vi "Get Log File Archive Location.vi"(8 "error in (no error)":errorcluster, 11 "log file in":T1 format="%.0x") -> (0 "error out":errorcluster, 1 "archive directory parts":string[](array[string]), 2 "archive closed log files":bool, 3 "log file out":T1 format="%.0x")   [LabVIEW 2027, in "Embedded Data Logger Scripting.lvlib"]
uses:
  Embedded Data Logger Scripting.lvlib
  <vilib>/NI VeriStand/Custom Device API/Custom Device Item Ref.ctl
  Shared/Constants.vi
  <vilib>/NI VeriStand/Custom Device API/Get Item Property (Boolean).vi
  <vilib>/NI VeriStand/Custom Device API/Get Item Property (String Array).vi
  <vilib>/NI VeriStand/Custom Device API/Custom Device API.lvlib
  Shared/Embedded Data Logger Shared.lvlib
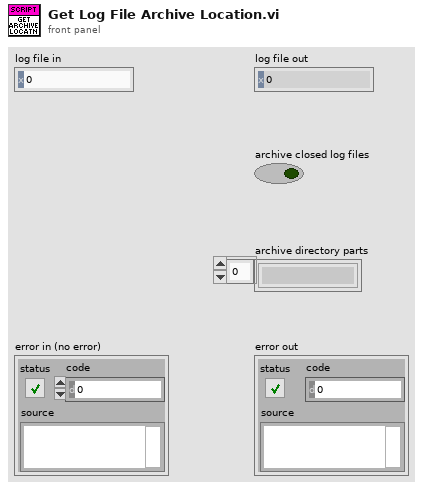
[diagram p1: front panel]
types:
  T1 = typedef "Custom Device API.lvlib/Custom Device Item Ref.ctl" = u64
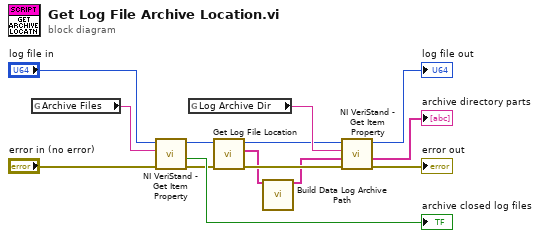
[diagram p0: block diagram]
diagram:
  n1 = global read "Constants.vi" "Archive Files"() -> (w7:string)
  n2 = call-poly <vilib>:"NI VeriStand - Get Item Property.vi"("error in (no error)"="error in (no error)", "Property Name"=w7, "Item Ref in"="log file in") -> ("error out"=w6:errorcluster, "Value"=→"archive closed log files":bool, "Item Ref out"=w5:T1)  [unwired: 1 in, 5 out]
  n3 = global read "Constants.vi" "Log Archive Dir"() -> (w14:string)
  n4 = call "Get Log File Location.vi"("error in (no error)"=w6, "log file in"=w5) -> ("error out"=w3:errorcluster, "directory parts"=w2:string[], "log file out"=w4:T1)  [unwired: 4 in, 3 out]
  n5 = call "Build Data Log Archive Path.vi"("Log Directory String Array"=w2) -> ("Log Archive Directory String Array"=w1:string[])  [unwired: 14 in]
  n6 = call-poly <vilib>:"NI VeriStand - Get Item Property.vi"("error in (no error)"=w3, "Default Value"=w1, "Property Name"=w14, "Item Ref in"=w4) -> ("error out"=→"error out":errorcluster, "Value"=→"archive directory parts":string[], "Item Ref out"=→"log file out":T1)  [unwired: 5 out]
